vi "Constants.vi"() -> ()   [LabVIEW 2026, in "Runtime Configuration Support Example Shared.lvlib"]
doc: "Use this Global VI to access the GUIDs assigned to the page resources of the Custom Device."
uses:
  Runtime Configuration Support Example Shared.lvlib
panel:
  in  "Tab Control":enum32{"GUIDs", "Constants", "Properties"}(tab)
  in  "Runtime Configuration Support Example":string="9c50e764-8e21-40d4-9c84-c31c997b404b"
  in  "Compiled.Settings":string="Compiled.Settings"
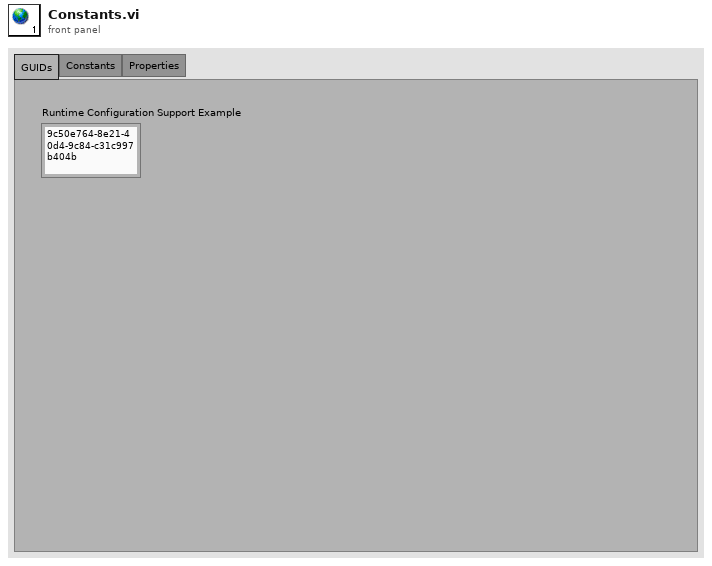
[diagram p1: front panel]
diagram:
